vi "Actor Core.vi"(8 "error in":errorcluster, 11 "Tiff Writer in":refnum<class "Tiff Writer.lvclass">) -> (0 "error out":errorcluster, 3 "Actor out":refnum<class "Actor.lvclass">)   [LabVIEW 2015, in "Tiff Writer.lvlib" / "Tiff Writer.lvclass"]
doc: "(<B>Filename</B>: Actor Framework.lvlib:Actor.lvclass:Actor Core.vi)\n\nReceives messages to the actor, reacts to them, and initiates any error handling that may shut the actor down.\n\nDescendant classes may override this VI to append parallel tasks for the actor to complete while it handles messages. Overrides use the Call Parent Method node."
uses:
  Tiff Writer.lvclass
  <vilib>/ActorFramework/Actor/Actor.lvclass
  BinaryTIFF/Class/TIFF.lvclass
  <vilib>/ActorFramework/Stop Msg/Stop Msg.lvclass
  BinaryTIFF v0.3.2/CLib/DCIMG2TIFF/DCIMG2TIFF.dll
  Resources/GLOBAL/GLOBAL Time-critical.vi
panel:
  in  "Stop Button":bool
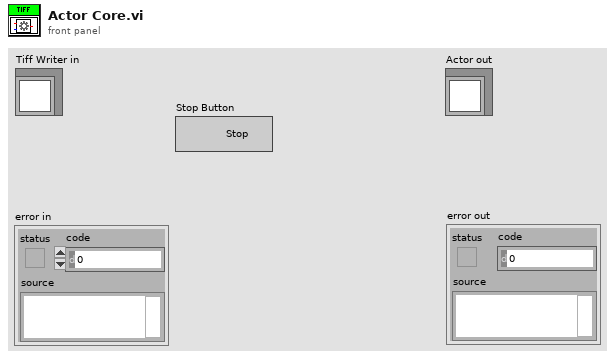
[diagram p1: front panel]
types:
  T1 = cluster{"Number of Frames":u32, "Image Width (px)":u32, "Image Height (px)":u32, "Pixel Size (nm)":dbl, "Exposure Time (ms)":dbl, "Frame Time (ms)":dbl, "Number of Channels":u32, "Camera Type":enum16{"<unknown>", "Evolve 512", "Orca-Flash 4.0 V2"}, "Bit Depth":u32, "Image Description":string}
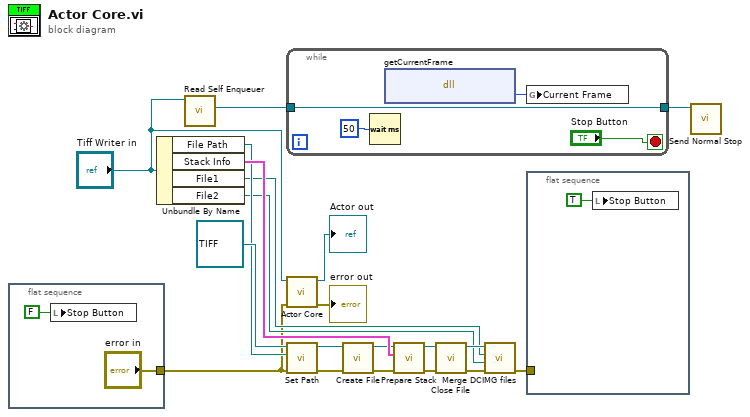
[diagram p0: block diagram]
diagram:
  n1 = flat-sequence {
    tunnel: ["error in"] -> w7
    frame #0 {
      n2 = local write "Stop Button"(FALSE ("Stop Button")) -> ()
    }
  }
  n3 = Unbundle By Name("Tiff Writer in") -> ("File Path"=w11:path, "Stack Info"=w15:T1, "File1"=w9:path, "File2"=w8:path)
  n4 = call <vilib>:"Read Self Enqueuer.vi"("Actor"="Tiff Writer in") -> ("Self Enqueuer"=w5:refnum<class "Message Enqueuer.lvclass">)  [unwired: 10 in]
  n5 = while {
    tunnel: [w24] -> w4
    tunnel: w5 -> [w24]
    stop <- "Stop Button" stop-if-true
    n6 = Wait (ms)(milliseconds to wait=u32 50) -> ()  [unwired: 1 out]
    n7 = dll-call lib="C:/LV/BinaryTIFF v0.3.2/CLib/DCIMG2TIFF/DCIMG2TIFF.dll" fn="getCurrentFrame"() -> ("Current Frame"=w23:u64)  [unwired: 3 in, 2 out]
    n8 = global write "GLOBAL Time-critical.vi" "Current Frame"(w23) -> ()
  }
  n9 = call-parent "Actor Core.vi"("error in"=w7, "Actor in"="Tiff Writer in") -> ("error out"=→"error out":errorcluster, "Actor out"=→"Actor out":refnum<class "Actor.lvclass">)  [unwired: 8 in]
  n10 = call-dynamic "Set Path.vi"("error in (no error)"=w7, "File Path"=w11, "TIFF in"=refnum<class "TIFF.lvclass"> refnum) -> ("error out"=w1:errorcluster, "TIFF out"=w12:refnum<class "TIFF.lvclass">)  [unwired: 7 in]
  n11 = call-dynamic "Create File.vi"("error in (no error)"=w1, "TIFF in"=w12) -> ("error out"=w14:errorcluster, "TIFF out"=w13:refnum<class "TIFF.lvclass">)  [unwired: 8 in]
  n12 = call-dynamic "Prepare Stack.vi"("error in (no error)"=w14, "Stack Info"=w15, "TIFF in"=w13) -> ("error out"=w17:errorcluster, "TIFF out"=w16:refnum<class "TIFF.lvclass">)  [unwired: 7 in]
  n13 = call-dynamic "Close File.vi"("error in (no error)"=w17, "TIFF in"=w16) -> ("error out"=w6:errorcluster, "TIFF out"=w10:refnum<class "TIFF.lvclass">)  [unwired: 8 in]
  n14 = call-dynamic "Merge DCIMG files.vi"("error in (no error)"=w6, "DCIMG Path 2"=w8, "DCIMG Path 1"=w9, "TIFF in"=w10) -> ("error out"=w3:errorcluster)  [unwired: 6 in, 1 out]
  n15 = flat-sequence {
    tunnel: w3 -> [_]
    frame #0 {
      n16 = local write "Stop Button"(TRUE ("Stop Button")) -> ()
    }
  }
  n17 = call <vilib>:"Send Normal Stop.vi"("Message Enqueuer"=w4) -> ()  [unwired: 10 in, 1 out]
